vi "Excel Easy Table.vi"   [LabVIEW 2020, in "NI_ReportGenerationToolkit.lvlib"]
doc: "Inserts and formats a table into a Microsoft Excel report. The data type you wire to the <B>text data</B> input determines the polymorphic instance to use."
uses:
  <vilib>/addons/_office/NI_ReportGenerationToolkit.lvlib
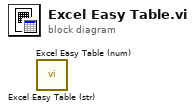
[diagram p0: block diagram]
diagram:
  n1 = call <vilib>:"Excel Easy Table (str).vi"() -> ()  [unwired: 11 in, 5 out]
  n2 = call <vilib>:"Excel Easy Table (num).vi"() -> ()  [unwired: 11 in, 5 out]
